vi "Param_init.vi"(4 "ParamTable":string="par_3", 6 "conninfo":T1={"host"="localhost", "port"="5432", "client_encoding"="WIN1251", "dbname"="data", "user"="postgres", "password"=""}, 7 "N_param":i32, 8 "error in (no error)":errorcluster, 9 "Names def":string[][](array[string]), 10 "Parameters def":dbl[][](array[numeric]), 11 "Parameters":string[](array[string])) -> (0 "error":errorcluster, 3 "Param out":T2)   [LabVIEW 2019, in "Inputs.lvlib"]
uses:
  Inputs.lvlib
  Ctl/Param.ctl
  Database/ctl/Coninfo.ctl
  Database/PostgreSQL.lvlib
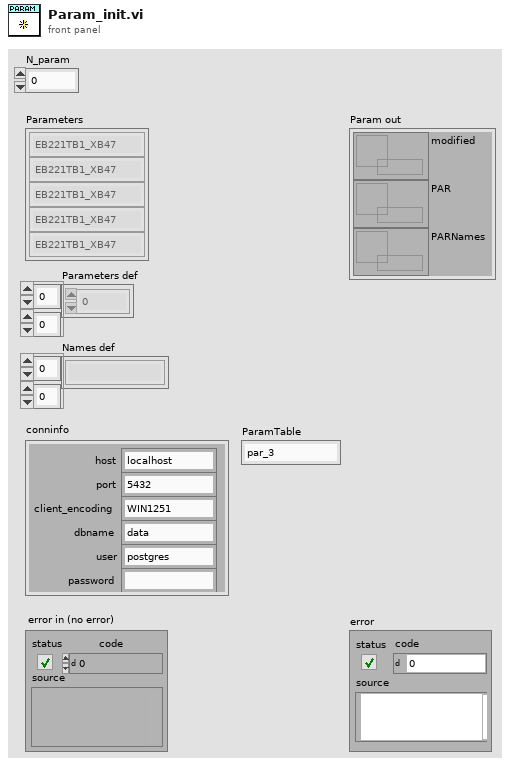
[diagram p1: front panel]
types:
  T1 = typedef "PostgreSQL.lvlib/Coninfo.ctl" = cluster{"host":string, "port":string, "client_encoding":string, "dbname":string, "user":string, "password":string}
  T2 = typedef "Inputs.lvlib/Param.ctl" = cluster{"modified":refnum<data-value>, "PAR":refnum<data-value>, "PARNames":refnum<data-value>}
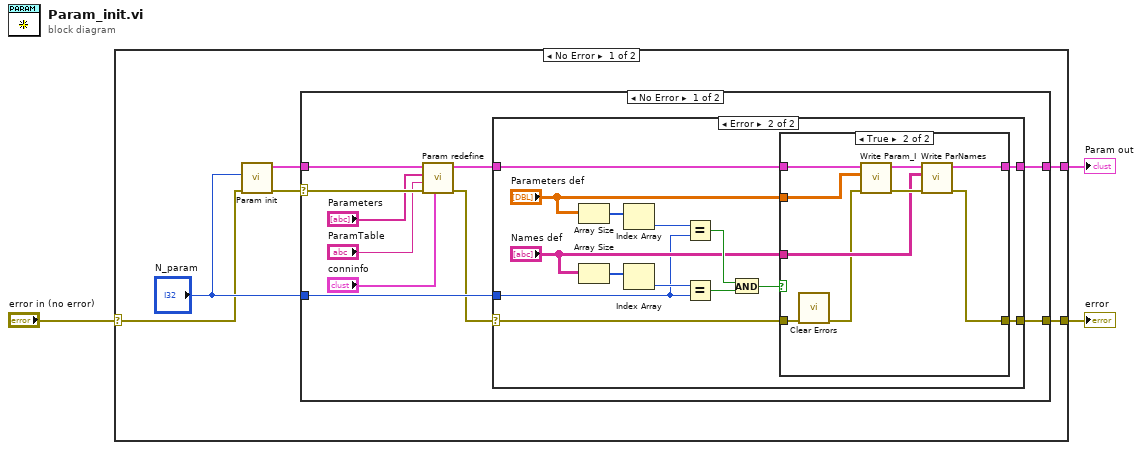
[diagram p0: block diagram]
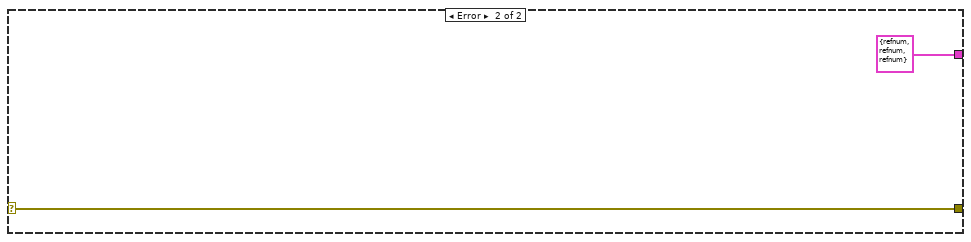
[diagram p5: hidden frame]
diagram:
  n1 = case shown="No Error" "error in (no error)" {
    selector: "error in (no error)" -> [w4 w50]
    tunnel: [w9 w50] -> w3
    tunnel: [w5 T2 {"modified"=refnum, "PAR"=refnum, "PARNames"=refnum} ("Param")] -> w2
    frame No Error {
      n2 = call "Param init.vi"("error in (no error)"=w4, "N_param"="N_param") -> ("error"=w6:errorcluster, "Param"=w7:T2)  [unwired: 8 in]
      n3 = case shown="No Error" w6 {
        selector: w6 -> [w16 w48]
        tunnel: "N_param" -> [w18 _]
        tunnel: [w19 w48] -> w9
        tunnel: w7 -> [w15 w47]
        tunnel: [w17 w47] -> w5
        frame No Error {
          n4 = call "Param redefine.vi"("conninfo"="conninfo", "error in (no error)"=w16, "ParamTable"="ParamTable", "Parameters"="Parameters", "Param in"=w15) -> ("error"=w13:errorcluster, "Param out"=w14:T2)  [unwired: 5 in]
          n5 = case shown="Error" w13 {
            selector: w13 -> [w21 w26]
            tunnel: [w21 w27] -> w19
            tunnel: w18 -> [_ w28]
            tunnel: w14 -> [w20 w23]
            tunnel: [w20 w22] -> w17
            frame No Error {
            }
            frame Error {
              n6 = Array Size(array="Parameters def") -> (size(s)=w30:i32[])
              n7 = Array Size(array="Names def") -> (size(s)=w31:i32[])
              n8 = Index Array(array=w30) -> (element=w32:i32)  [unwired: 1 in]
              n9 = Index Array(array=w31) -> (element=w33:i32)  [unwired: 1 in]
              n10 = Equal?(x=w32, y=w28) -> (x = y?=w34:bool)
              n11 = Equal?(x=w33, y=w28) -> (x = y?=w35:bool)
              n12 = And(x=w34, y=w35) -> (x .and. y?=w24:bool)
              n13 = case shown="True" w24 {
                tunnel: "Parameters def" -> [_ w43]
                tunnel: "Names def" -> [_ w42]
                tunnel: [w36 w41] -> w27
                tunnel: w26 -> [w36 w39]
                tunnel: w23 -> [w37 w44]
                tunnel: [w37 w40] -> w22
                frame False {
                }
                frame True {
                  n14 = call <vilib>:"Clear Errors.vi"("error in (no error)"=w39) -> ("error out"=w38:errorcluster)  [unwired: 5 in, 1 out]
                  n15 = call "Write Param_I.vi"("error in (no error)"=w38, "Param"=w43, "Param in"=w44) -> ("error out"=w45:errorcluster, "Param out"=w46:T2)  [unwired: 7 in]
                  n16 = call "Write ParNames.vi"("error in (no error)"=w45, "PARNames"=w42, "Param in"=w46) -> ("error out"=w41:errorcluster, "Param out"=w40:T2)  [unwired: 7 in]
                }
              }
            }
          }
        }
        frame Error {
        }
      }
    }
    frame Error {
    }
  }
  "Param out" <- w2
  "error" <- w3
